vi "Toggle.vi"(1 "In":bool) -> (0 "Toggled Output":bool)   [LabVIEW 2025]
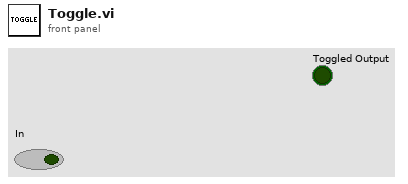
[diagram p1: front panel]
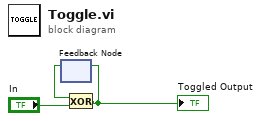
[diagram p0: block diagram]
diagram:
  n1 = feedback #1() -> (w1:bool)  [unwired: 1 in]
  n2 = Exclusive Or(1:"In", 2:w1) -> (0:w2:bool)
  "Toggled Output" <- w2
  n3 = feedback-in #1(w2) -> ()
